vi "update-ExpgroupSD.vi"(2 "error in":errorcluster, 3 "String File Paths":string[](array[string]), 4 "EXP group":refnum<class "Experiments_group.lvclass">) -> (0 "error out":errorcluster, 1 "EXP group out":refnum<class "Experiments_group.lvclass">)   [LabVIEW 2015]
uses:
  Classes/Experiments_group.lvclass
  Classes/Experiment.lvclass
  <vilib>/Utility/file.llb/Read Delimited Spreadsheet (DBL).vi
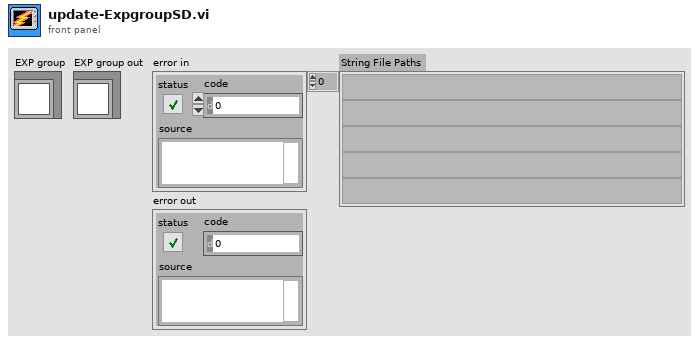
[diagram p1: front panel]
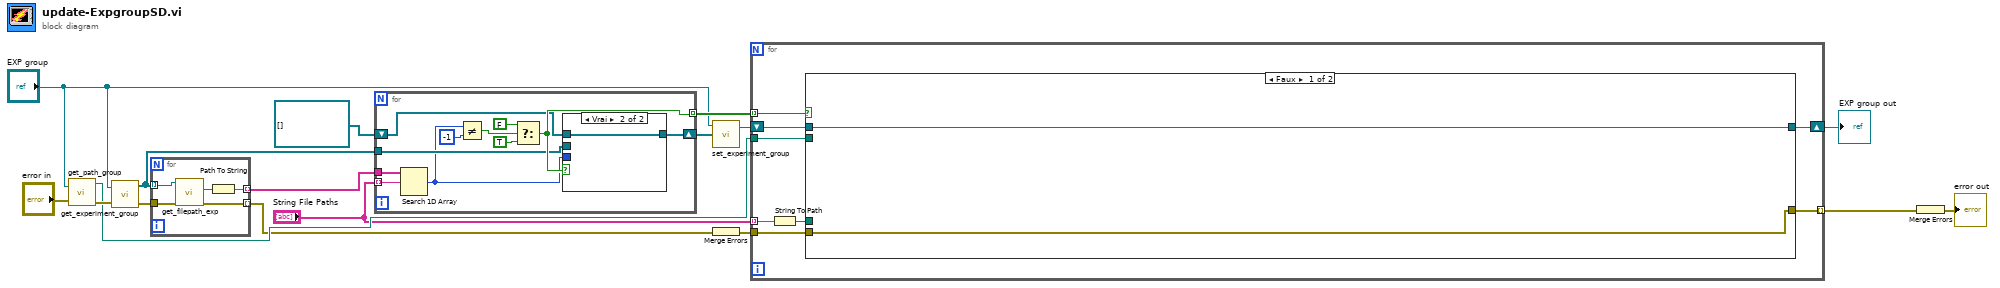
[diagram p0: block diagram]
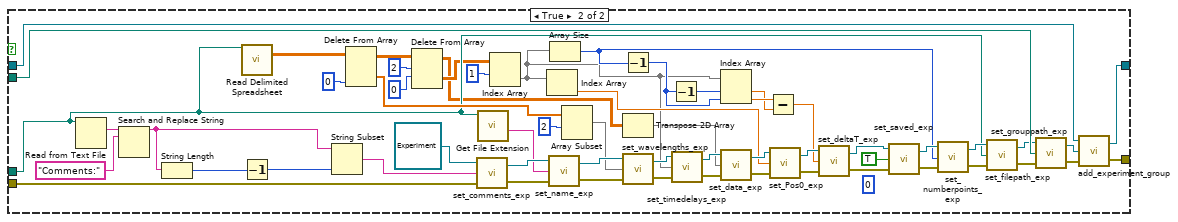
[diagram p2: hidden frame]
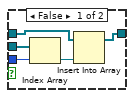
[diagram p3: hidden frame]
diagram:
  n1 = call-dynamic "get_path_group.vi"("Experiments_group.lvclass in"="EXP group", "error in (no error)"="error in") -> ("Path"=w13:path, "error out"=w14:errorcluster)  [unwired: 1 out]
  n2 = call-dynamic "get_experiment_group.vi"("Experiments_group.lvclass in"="EXP group", "error in (no error)"=w14) -> ("Experiments"=w4:refnum<class "Experiment.lvclass">[], "error out"=w17:errorcluster)  [unwired: 1 out]
  n3 = for {
    tunnel: w4 -> [w22] mode=indexing
    tunnel: w17 -> [w21]
    tunnel: [w20] -> w11 mode=indexing
    tunnel: [w19] -> w16 mode=indexing
    n4 = call-dynamic "get_filepath_exp.vi"("error in (no error)"=w21, "Experiment.lvclass in"=w22) -> ("error out"=w20:errorcluster, "FilePath"=w18:path)  [unwired: 7 in, 1 out]
    n5 = Path To String(path=w18) -> (string=w19:string)
  }
  n6 = for {
    tunnel: "String File Paths" -> [w28] mode=indexing
    tunnel: w16 -> [w29]
    tunnel: [w27] -> w8 mode=indexing
    tunnel: w4 -> [w26]
    shift-right: [w23] -> w2
    shift-left: refnum<class "Experiment.lvclass">[] [] ("Experiments") -> [w24]
    n7 = Search 1D Array(1D array=w29, element=w28) -> (index of element=w25:i32)  [unwired: 1 in]
    n8 = Not Equal?(x=w25, y=-1) -> (x != y?=w32:bool)
    n9 = Select(t=FALSE, s=w32, f=TRUE) -> (s? t:f=w27:bool)
    n10 = case shown="Vrai" w27 {
      tunnel: w26 -> [w38 _]
      tunnel: w25 -> [w37 _]
      tunnel: w24 -> [w35 w39]
      tunnel: [w34 w39] -> w23
      frame False {
        n11 = Index Array(array=w38, index=w37) -> (element=w36:refnum<class "Experiment.lvclass">)
        n12 = Insert Into Array(array=w35, new element=w36) -> (w34:refnum<class "Experiment.lvclass">[])  [unwired: 1 in]
      }
      frame True {
      }
    }
  }
  n13 = call-dynamic "set_experiment_group.vi"("Experiments"=w2, "Experiments_group.lvclass in"="EXP group") -> ("Experiments_group.lvclass out"=w1:refnum<class "Experiments_group.lvclass">)  [unwired: 1 in, 1 out]
  n14 = Merge Errors(w11) -> (w10:errorcluster)
  n15 = for {
    tunnel: w8 -> [w47] mode=indexing
    tunnel: w13 -> [w46]
    shift-right: [w44] -> w12
    shift-left: w1 -> [w45]
    tunnel: [w43] -> w6 mode=indexing
    tunnel: w10 -> [w42]
    tunnel: "String File Paths" -> [w41] mode=indexing
    n16 = String To Path(string=w41) -> (path=w40:path)
    n17 = case shown="Faux" w47 {
      tunnel: w40 -> [_ w60]
      tunnel: w46 -> [_ w106]
      tunnel: w45 -> [w49 w103]
      tunnel: [w49 w102] -> w44
      tunnel: [w48 w101] -> w43
      tunnel: w42 -> [w48 w100]
      frame False {
      }
      frame True {
        (unwired) 0 ("index")
        n18 = Read from Text File(file (use dialog)=w60) -> (text=w80:string)  [unwired: 3 in, 3 out]
        n19 = Search and Replace String(input string=w80, search string="Comments:") -> (result string=w53:string)  [unwired: 6 in, 3 out]
        n20 = String Length(string=w53) -> (length=w52:i32)
        n21 = call-poly <vilib>:"Read Delimited Spreadsheet.vi"("file path (dialog if empty)"=w60) -> ("all rows"=w75:dbl[][])  [unwired: 9 in, 5 out]
        n22 = Decrement(x=w52) -> (x-1=w51:i32)
        n23 = String Subset(string=w53, length (rest)=w51) -> (substring=w50:string)  [unwired: 1 in]
        n24 = Delete From Array(array=w75, index (col)=0 ("disabled index (col)")) -> (deleted portion=w73:dbl[], array with subset deleted=w74:dbl[][])  [unwired: 2 in]
        n25 = Delete From Array(array=w74, length=2, index (row)=0) -> (deleted portion=w58:dbl[][], array with subset deleted=w56:dbl[][])  [unwired: 1 in]
        n26 = call-dynamic "set_comments_exp.vi"("error in (no error)"=w100, "Comments"=w50, "Experiment.lvclass in"=refnum<class "Experiment.lvclass"> refnum ("Experiment.lvclass")) -> ("error out"=w99:errorcluster, "Experiment.lvclass out"=w78:refnum<class "Experiment.lvclass">)
        n27 = call <vilib>:"Get File Extension.vi"("file"=w60) -> ("filename without extension"=w77:string)  [unwired: 6 in, 4 out]
        n28 = Index Array(array=w58, index (row)=1) -> (element=w57:dbl[])  [unwired: 1 in]
        n29 = Index Array(array=w57) -> (element=w68:dbl)  [unwired: 1 in]
        n30 = call-dynamic "set_name_exp.vi"("error in (no error)"=w99, "Exp name"=w77, "Experiment.lvclass in"=w78) -> ("error out"=w98:errorcluster, "Experiment.lvclass out"=w76:refnum<class "Experiment.lvclass">)
        n31 = Array Size(array=w57) -> (size(s)=w61:i32)
        n32 = Array Subset(array=w73, index=2) -> (w70:dbl[])  [unwired: 1 in]
        n33 = Decrement(x=w61) -> (x-1=w67:i32)
        n34 = Transpose 2D Array(2D array=w56) -> (transposed array=w55:dbl[][])
        n35 = call-dynamic "set_wavelengths_exp.vi"("error in (no error)"=w98, "wavelengths"=w70, "Experiment.lvclass in"=w76) -> ("error out"=w89:errorcluster, "Experiment.lvclass out"=w97:refnum<class "Experiment.lvclass">)
        n36 = Decrement(x=w67) -> (x-1=w66:i32)
        n37 = call-dynamic "set_timedelays_exp.vi"("error in (no error)"=w89, "timedelays"=w57, "Experiment.lvclass in"=w97) -> ("error out"=w88:errorcluster, "Experiment.lvclass out"=w96:refnum<class "Experiment.lvclass">)
        n38 = Index Array(array=w57, index #1=w66, index #2=w67) -> (element #1=w64:dbl, element #2=w65:dbl)
        n39 = call-dynamic "set_data_exp.vi"("error in (no error)"=w88, "Data"=w55, "Experiment.lvclass in"=w96) -> ("error out"=w87:errorcluster, "Experiment.lvclass out"=w95:refnum<class "Experiment.lvclass">)
        n40 = Subtract(x=w65, y=w64) -> (x-y=w63:dbl)
        n41 = call-dynamic "set_Pos0_exp.vi"("error in (no error)"=w87, "Pos0,ps"=w68, "Experiment.lvclass in"=w95) -> ("error out"=w86:errorcluster, "Experiment.lvclass out"=w94:refnum<class "Experiment.lvclass">)
        n42 = call-dynamic "set_deltaT_exp.vi"("error in (no error)"=w86, "deltaTlast"=w63, "Experiment.lvclass in"=w94) -> ("error out"=w85:errorcluster, "Experiment.lvclass out"=w93:refnum<class "Experiment.lvclass">)
        n43 = call-dynamic "set_saved_exp.vi"("error in (no error)"=w85, "Saved"=TRUE, "Experiment.lvclass in"=w93) -> ("error out"=w84:errorcluster, "Experiment.lvclass out"=w92:refnum<class "Experiment.lvclass">)
        n44 = call-dynamic "set_numberpoints_exp.vi"("error in (no error)"=w84, "numberpoints"=w61, "Experiment.lvclass in"=w92) -> ("error out"=w83:errorcluster, "Experiment.lvclass out"=w91:refnum<class "Experiment.lvclass">)
        n45 = call-dynamic "set_filepath_exp.vi"("error in (no error)"=w83, "FilePath"=w60, "Experiment.lvclass in"=w91) -> ("error out"=w82:errorcluster, "Experiment.lvclass out"=w90:refnum<class "Experiment.lvclass">)
        n46 = call-dynamic "set_grouppath_exp.vi"("error in (no error)"=w82, "GroupPath"=w106, "Experiment.lvclass in"=w90) -> ("error out"=w105:errorcluster, "Experiment.lvclass out"=w104:refnum<class "Experiment.lvclass">)
        n47 = call-dynamic "add_experiment_group.vi"("error in (no error)"=w105, "Experiment.lvclass"=w104, "Experiments_group.lvclass in"=w103) -> ("error out"=w101:errorcluster, "Experiments_group.lvclass out"=w102:refnum<class "Experiments_group.lvclass">)
      }
    }
  }
  "EXP group out" <- w12
  n48 = Merge Errors(w6) -> (→"error out":errorcluster)
